vi "File Controller_Create.vi"(0 "reference in":refnum<class "File Controller.lvclass">, 5 "error in (no error)":errorcluster) -> (14 "reference out":refnum<class "File Controller.lvclass">, 19 "error out":errorcluster)   [LabVIEW 2015, in "File Controller.lvclass"]
doc: "Constructor."
uses:
  File Controller.lvclass
  <vilib>/addons/_AddQ/G#Object/G#Object.lvclass
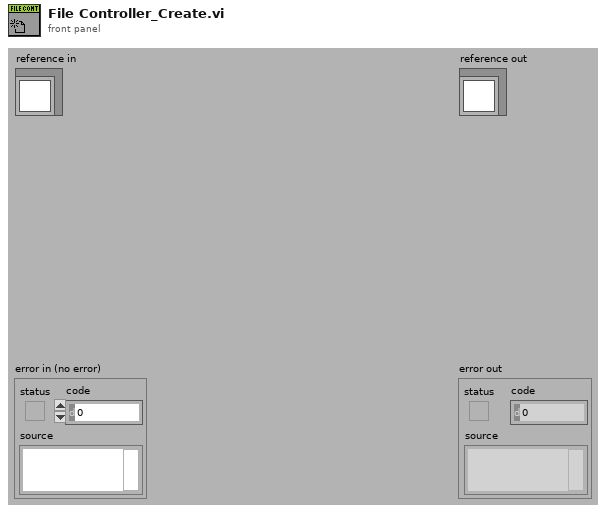
[diagram p1: front panel]
types:
  T1 = typedef "File Controller.lvclass/ClassAttributesRef.ctl" = refnum<data-value>
  T2 = typedef "File Controller.lvclass/ClassAttributes.ctl" = cluster{"Dummy":bool, "File Controller.lvclass":refnum<class "File Controller.lvclass">}
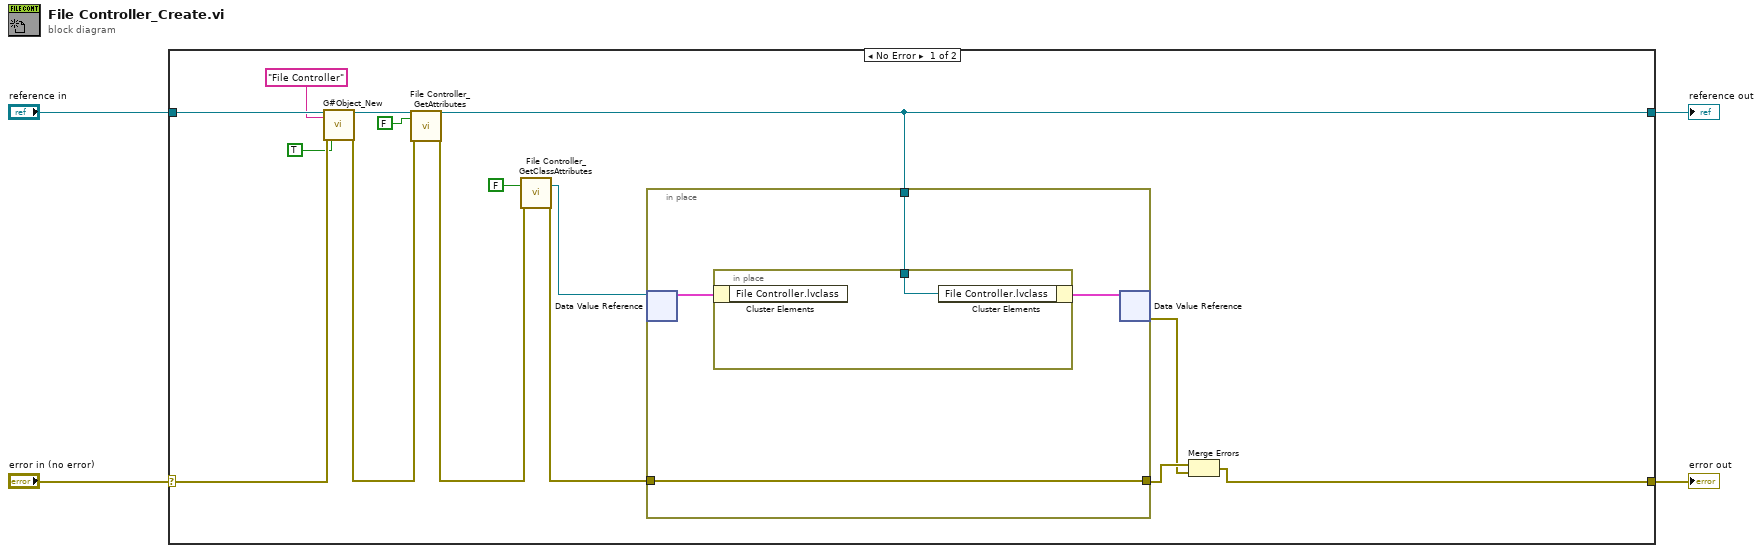
[diagram p0: block diagram]
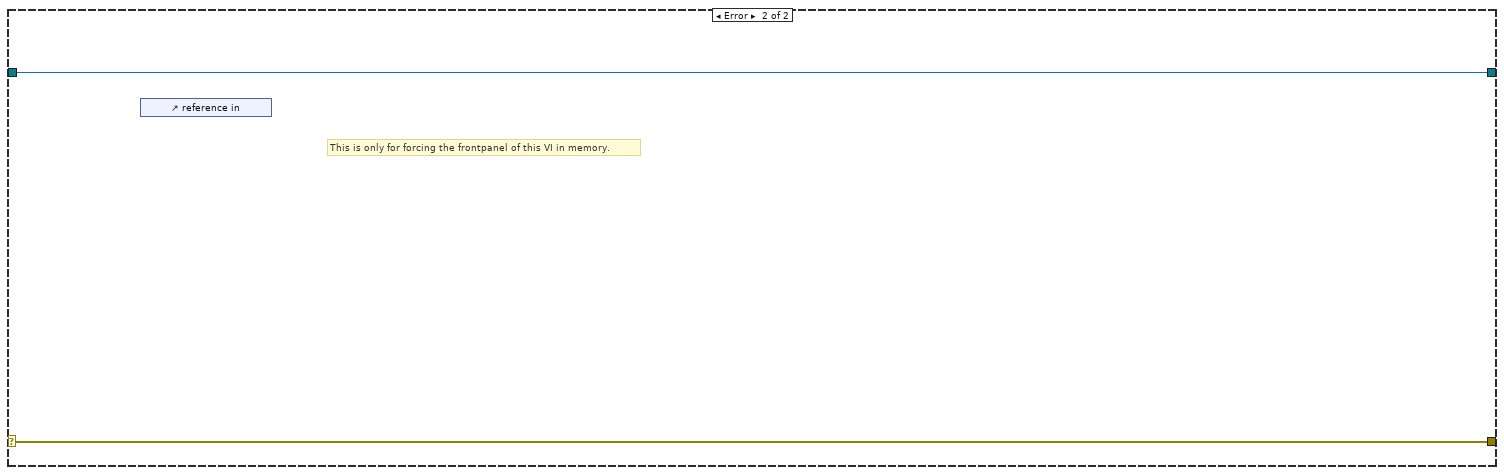
[diagram p2: hidden frame]
diagram:
  n1 = case shown="No Error" "error in (no error)" {
    selector: "error in (no error)" -> [w18 w26]
    tunnel: [w5 w26] -> w3
    tunnel: [w6 w25] -> w1
    tunnel: "reference in" -> [w19 w25]
    frame No Error {
      n2 = call <vilib>:"G#Object_New.vi"("reference in"=w19, "object name"="File Controller", "error in (no error)"=w18, "user counter (T)?"=TRUE ("User Counter")) -> ("reference out"=w14:refnum<class "File Controller.lvclass">, "error out"=w13:errorcluster)  [unwired: 13 in, 1 out]
      n3 = call "File Controller_GetAttributes.vi"("reference in"=w14, "return data? (T)"=FALSE ("return data"), "error in (no error)"=w13) -> ("reference out"=w6:refnum<class "File Controller.lvclass">, "error out"=w11:errorcluster)  [unwired: 13 in, 2 out]
      n4 = call "File Controller_GetClassAttributes.vi"("return data? (T)"=FALSE, "error in (no error)"=w11) -> ("class attributes ref"=w9:T1, "error out"=w10:errorcluster)  [unwired: 14 in, 2 out]
      n5 = in-place {
        in-place-border: w10 -> [w21]
        in-place-border: [w21] -> w16
        in-place-border: w6 -> [w20]
        n6 = in-place-dvr #1(w9) -> (w22:T2)  [unwired: 1 out]
        n7 = in-place {
          in-place-border: w20 -> [w24]
          n8 = in-place-cluster #2(w22) -> ()  [unwired: 1 out]
          n9 = in-place-cluster #2("File Controller.lvclass"=w24) -> (w23:T2)
        }
        n10 = in-place-dvr #1(w23) -> (w15:errorcluster)  [unwired: 1 out]
      }
      n11 = Merge Errors(w16, w15) -> (w5:errorcluster)
    }
    frame Error {
      # "This is only for forcing the frontpanel of this VI in memory."
      n12 = control-ref of="reference in"() -> ()  [unwired: 1 out]
    }
  }
  "error out" <- w3
  "reference out" <- w1
